vi "Write Or Not.vi"(1 "Time":timestamp, 3 "data in":variant) -> (0 "Write?":bool)   [LabVIEW 2019, in "Logger.PGSQL.lvlib" / "Logger.PGSQL.lvclass"]
uses:
  Logger.PGSQL.lvclass
  <userlib>/LevyLab/LV-Data/LV-Data.PG/LV-Data.PGSQL.lvclass
  <vilib>/Utility/Data Type/NI_Data Type.lvlib
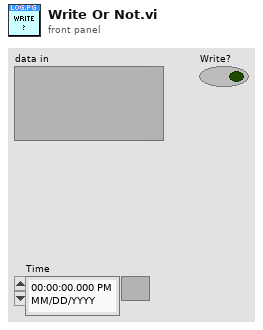
[diagram p1: front panel]
types:
  T1 = typedef "NI_Data Type.lvlib/Data Type.ctl" = enum8{"Invalid Type", "Void", "I8", "I16", "I32", "I64", "U8", "U16", "U32", "U64", "Single Float", "Double Float", "Extended Float", "Single Complex", "Double Complex", "Extended Complex", "Enum U8", "Enum U16", "Enum U32", "Enum U64", "Single Float With Unit", "Double Float With Unit", "Extended Float With Unit", "Single Complex with Unit", "Double Complex with Unit", "Extended Complex with Unit", "Boolean", "String", "Path", "Picture", "Tag", "Array", "Cluster", "Variant", "LV Variant", "Waveform", "Timestamp", "Digital Waveform", "Digital Data", "ExpressData", "Refnum", "External Data", "VI", "Poly VI", "LabVIEW Class Instance", "Fixed Point", "Set Collection", "Map Collection"}
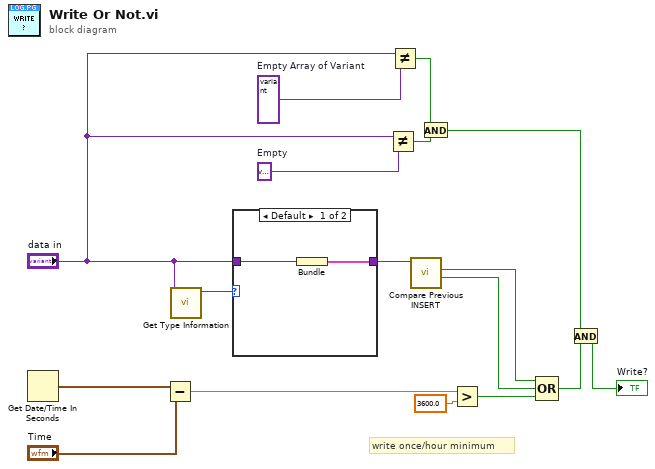
[diagram p0: block diagram]
diagram:
  w2 = variant(variant[] [])  # Empty Array of Variant
  w4 = variant  # Empty
  # "write once/hour minimum"
  n1 = Get Date/Time In Seconds() -> (seconds since 1Jan1904=w14:timestamp)
  n2 = Subtract(x=w14, y="Time") -> (x-y=w15:dbl)
  n3 = call <vilib>:"Get Type Information.vi"("variant"="data in") -> ("type"=w11:T1)  [unwired: 6 in, 4 out]
  n4 = case shown="Default" w11 {
    tunnel: "data in" -> [w19 w20]
    tunnel: [w18 w20] -> w10
    frame Default {
      n5 = Bundle("data in"=w19) -> (w18:cluster{"data in":variant})  [unwired: 1 in]
    }
    frame "Array", "Cluster" {
    }
  }
  n6 = Not Equal?(x="data in", y=w4) -> (x != y?=w8:bool)
  n7 = Not Equal?(x="data in", y=w2) -> (x != y?=w9:bool)
  n8 = call <userlib>:"Compare Previous INSERT.vi"("Data"=w10) -> ("Some Different"=w13:bool, "All Different"=w12:bool)  [unwired: 7 in, 2 out]
  n9 = And(x=w9, y=w8) -> (x .and. y?=w7:bool)
  n10 = Greater?(x=w15, y=3600.0) -> (0:w17:bool)
  n11 = Compound Arithmetic op=OR(w12, w13, w17) -> (w6:bool)
  n12 = And(x=w7, y=w6) -> (x .and. y?=→"Write?":bool)
